vi "SwerveHomeStore.vi"(6 "Update?":bool, 8 "RearRightHomeIn":dbl, 9 "RearLeftHomeIn":dbl, 10 "FrontRightHomeIn":dbl, 11 "FrontLeftHomeIn":dbl) -> (0 "RearRightHomeOut":dbl, 1 "RearLeftHomeOut":dbl, 2 "FrontRightHomeOut":dbl, 3 "FrontLeftHomeOut":dbl)   [LabVIEW 2018]
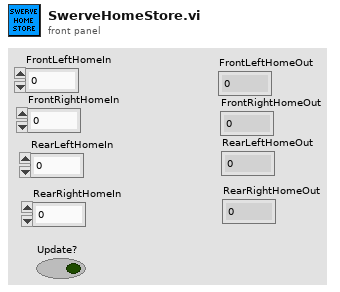
[diagram p1: front panel]
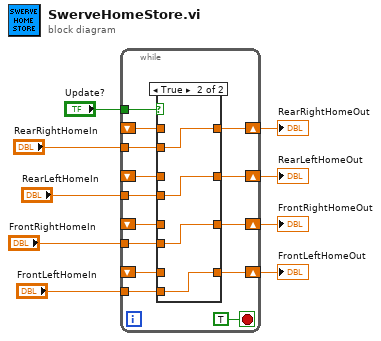
[diagram p0: block diagram]
diagram:
  n1 = while {
    tunnel: "Update?" -> [w22]
    tunnel: "FrontLeftHomeIn" -> [w21]
    tunnel: "FrontRightHomeIn" -> [w20]
    tunnel: "RearLeftHomeIn" -> [w19]
    tunnel: "RearRightHomeIn" -> [w18]
    shift-right: [w14] -> w4
    shift-left: _ -> [w13]
    shift-right: [w15] -> w3
    shift-left: _ -> [w12]
    shift-right: [w16] -> w2
    shift-left: _ -> [w11]
    shift-right: [w17] -> w1
    shift-left: _ -> [w10]
    stop <- TRUE stop-if-true
    n2 = case shown="True" w22 {
      tunnel: [w27 w31] -> w14
      tunnel: w21 -> [_ w31]
      tunnel: [w26 w30] -> w15
      tunnel: w20 -> [_ w30]
      tunnel: [w25 w29] -> w16
      tunnel: w19 -> [_ w29]
      tunnel: [w24 w28] -> w17
      tunnel: w18 -> [_ w28]
      tunnel: w13 -> [w27 _]
      tunnel: w12 -> [w26 _]
      tunnel: w11 -> [w25 _]
      tunnel: w10 -> [w24 _]
      frame False {
      }
      frame True {
      }
    }
  }
  "FrontLeftHomeOut" <- w4
  "FrontRightHomeOut" <- w3
  "RearRightHomeOut" <- w1
  "RearLeftHomeOut" <- w2
